vi "Exponential random numbers examples.vi"() -> ()   [LabVIEW 2010]
uses:
  <vilib>/Analysis/NI_AALBase.lvlib
panel:
  in  "Histogram intervals":i32=10
  out "Histogram":T1(graph)
  out "Waveform Graph\nof random numbers":dbl[](graph)
  in  "Desired Expected random number":dbl
  in  "Number of random numbers":i32
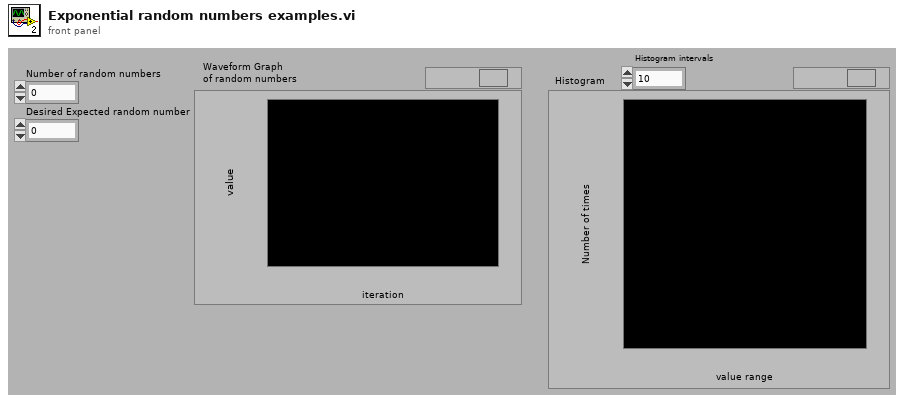
[diagram p1: front panel]
types:
  T1 = cluster{"X Values":dbl[], "Histogram: h(x)":i32[]}
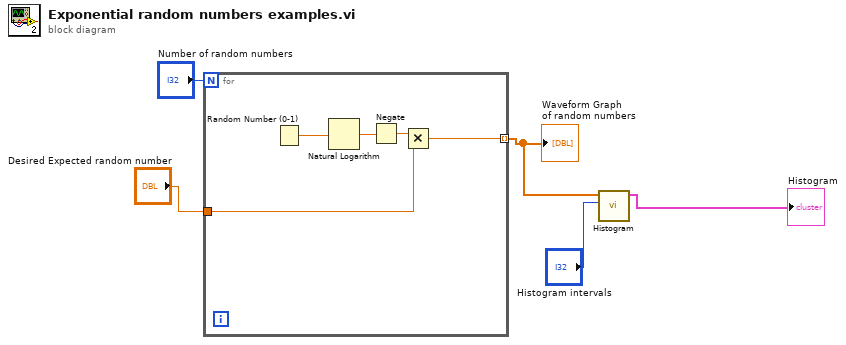
[diagram p0: block diagram]
diagram:
  n1 = for {
    N: "Number of random numbers" -> [_]
    tunnel: "Desired Expected random number" -> [w7]
    tunnel: [w6] -> w3 mode=indexing
    n2 = Random Number (0-1)() -> (number: 0 to 1=w10:dbl)
    n3 = Natural Logarithm(1:w10) -> (0:w9:dbl)
    n4 = Negate(x=w9) -> (-x=w8:dbl)
    n5 = Multiply(x=w8, y=w7) -> (x*y=w6:dbl)
  }
  "Waveform Graph\nof random numbers" <- w3
  n6 = call <vilib>:"Histogram.vi"("intervals"="Histogram intervals", "X"=w3) -> ("Histogram Graph"=→"Histogram":T1)  [unwired: 6 in, 3 out]
